vi "_Update Oscillators.vi"(4 "Pole In":bool[](array[boolean]), 5 "UpdateInput (F)":bool, 6 "ADC Array":i32[](array[numeric]), 7 "ADC Table":T1[](array[typedef]), 8 "Pole Swap (T)":bool=TRUE, 9 "Update (T)":bool=TRUE, 10 "Mode(pos)":bool=TRUE, 11 "Oscillator Settings":refnum<vi>) -> (1 "Q1RF Frequency":dbl, 3 "Pole":bool[](array[boolean]))   [LabVIEW 2012]
uses:
  Type/_RT Configuration 2.ctl
  Type/_RT Command.ctl
  Configuration/_Global Configuration.vi
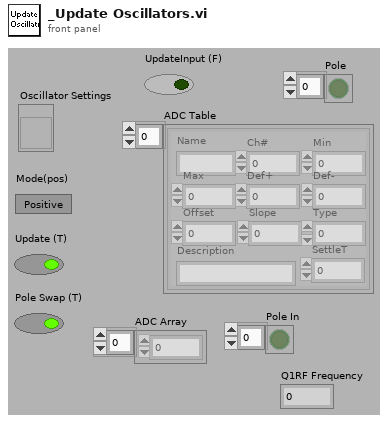
[diagram p1: front panel]
types:
  T1 = typedef "_RT Configuration 2.ctl" = cluster{"Name":string, "Ch#":u8, "Min":dbl, "Max":dbl, "Def+":dbl, "Def-":dbl, "Offset":dbl, "Slope":dbl, "Type":u8, "Description":string, "SettleT":dbl}
  T2 = typedef "_RT Instrument 2.ctl" = cluster{"Table":T1[], "Instrument":string[]}
  T3 = typedef "_RT Command.ctl" = enum16{"Start", "Stop", "Runtime Update", "Get Data", "Get Info", "Get Status", "Get Param", "Get Config", "Get Table", "Read ADC", "Set Oscillator", "Update Config", "Update Table", "Set All Pol", "Set Pol and DC", "Set Max Mass", "Toggle RP", "Toggle EL", "Set PIC", "Initialize Turbo", "Send Turbo Comm", "Close Turbo", "P1", "P2", "P3", "Send Serial", "Set LC Out", "Get LC In", "Read VAC", "Test Table", "Toggle Power", "Get Startup", "Set Startup", "Get ADC Table", "Set ADC Table", "Get Brief Status", "Get Detail Status", "Auxiliary Update", "Set CC Logics", "Set CC Input Logics", "Ignore Error"}
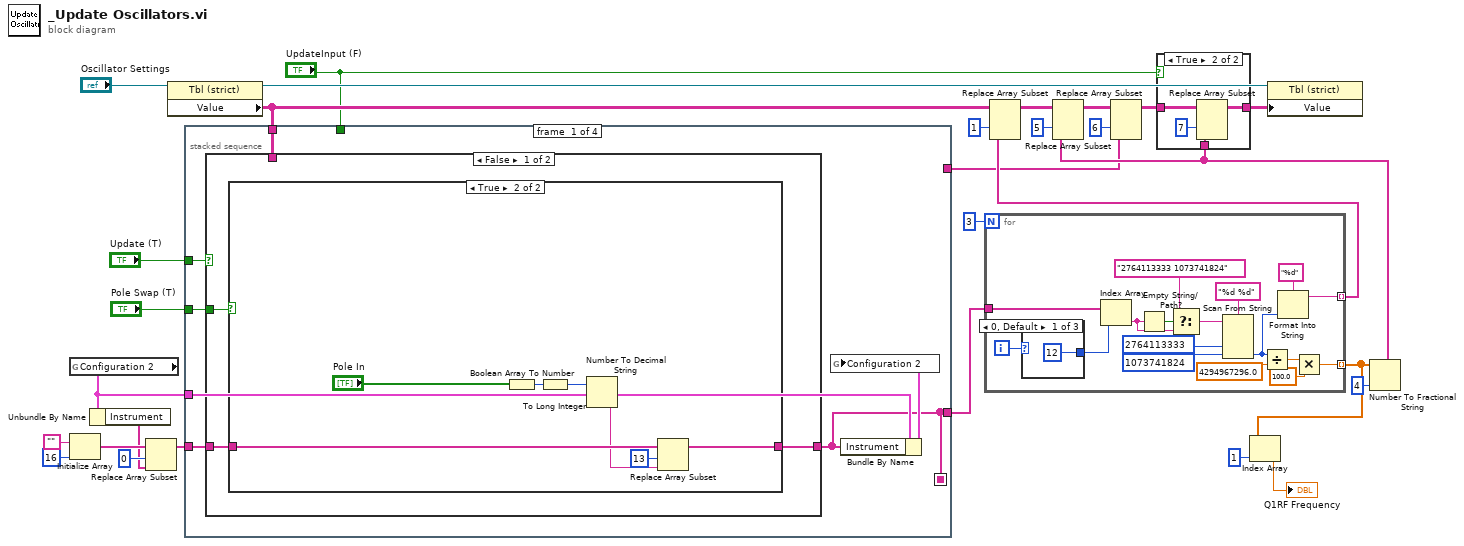
[diagram p0: block diagram]
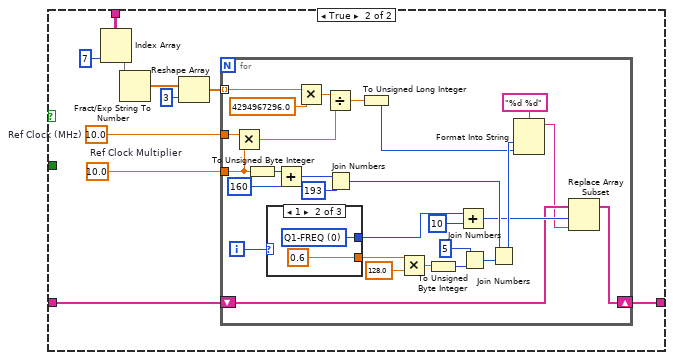
[diagram p4: hidden frame]
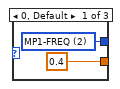
[diagram p5: hidden frame]
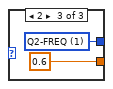
[diagram p6: hidden frame]
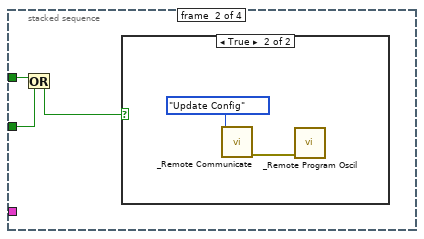
[diagram p7: hidden frame]
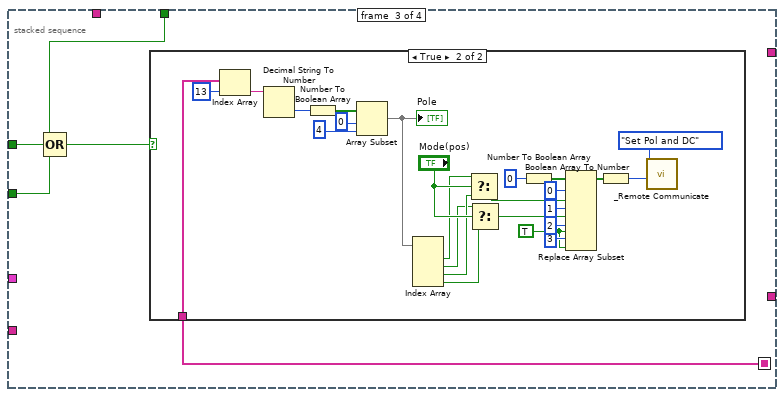
[diagram p9: hidden frame]
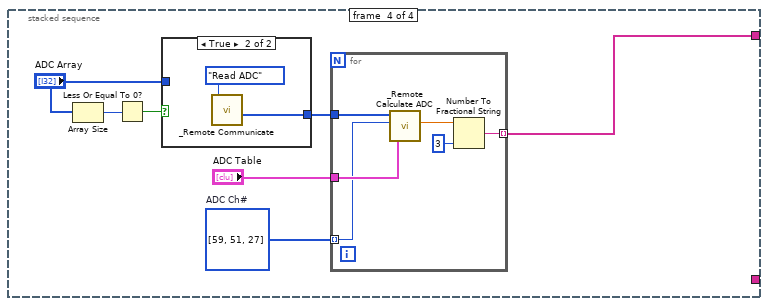
[diagram p11: hidden frame]
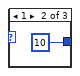
[diagram p13: hidden frame]
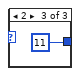
[diagram p14: hidden frame]
diagram:
  n1 = global read "_Global Configuration.vi" "Configuration 2"() -> (w22:T2)
  n2 = Initialize Array("", 16 ("dimension size")) -> (w26:string[])
  n3 = Unbundle By Name(w22) -> ("Instrument"=w24:string[])
  n4 = Replace Array Subset(array=w26, new element=w24, index=0) -> (w23:string[])
  n5 = property class="Tbl (strict)"(reference="Oscillator Settings") -> (reference out=w19:refnum<vi>, "Value"=w11:string[][])  [unwired: 1 in, 1 out]
  n6 = stacked-sequence {
    seq-local: [w30 _ _ _] -> [_ _ w101 _]
    tunnel: w11 -> [w36 _ _ _]
    tunnel: w23 -> [w35 _ _ _]
    tunnel: w22 -> [w33 _ _ _]
    tunnel: [w30 _ _ _] -> w13
    tunnel: "Update (T)" -> [w32 w94 w99 _]
    tunnel: "Pole Swap (T)" -> [w31 w93 w98 _]
    tunnel: [_ _ _ w130] -> w5
    tunnel: "UpdateInput (F)" -> [_ _ w100 _]
    frame #0 {
      n7 = case shown="False" w32 {
        tunnel: w36 -> [_ w57]
        tunnel: w35 -> [w39 w49]
        tunnel: [w37 w48] -> w30
        tunnel: w31 -> [w38 _]
        frame False {
          n8 = case shown="True" w38 {
            tunnel: w39 -> [w40 w45]
            tunnel: [w40 w44] -> w37
            frame False {
            }
            frame True {
              n9 = Boolean Array To Number(Boolean array="Pole In") -> (number=w46:u32)
              n10 = To Long Integer(number=w46) -> (32bit integer=w47:i32)
              n11 = Number To Decimal String(number=w47) -> (decimal integer string=w43:string)  [unwired: 1 out]
              n12 = Replace Array Subset(array=w45, new element=w43, index=13) -> (w44:string[])
            }
          }
        }
        frame True {
          w53 = 10.0  # Ref Clock Multiplier
          w54 = 10.0  # Ref Clock (MHz)
          n13 = Index Array(array=w57, index (col)=7 ("disabled index (col)")) -> (element=w55:string[])  [unwired: 1 in]
          n14 = Fract/Exp String To Number(string=w55) -> (number=w52:dbl[])  [unwired: 4 out]
          n15 = Reshape Array(w52, 3 ("dimension size")) -> (w51:dbl[])
          n16 = for {
            tunnel: w54 -> [w80]
            tunnel: w53 -> [w77]
            tunnel: w51 -> [w82] mode=indexing
            shift-right: [w58] -> w48
            shift-left: w49 -> [w60]
            i -> [w85]
            n17 = Multiply(x=w80, y=w77) -> (x*y=w79:dbl)
            n18 = To Unsigned Byte Integer(number=w77) -> (unsigned 8bit integer=w78:u8)
            n19 = case shown="1" w85 {
              tunnel: [w87 w89 w91] -> w62
              tunnel: [0.4 ("t") 0.6 ("t") 0.6 ("t")] -> w71
              frame 0, Default {
                w87 = u32 2 items=["Q1-FREQ", "Q2-FREQ", "MP1-FREQ"] ("Chip Select")
              }
              frame 1 {
                w89 = u32 0 items=["Q1-FREQ", "Q2-FREQ", "MP1-FREQ"] ("Chip Select")
              }
              frame 2 {
                w91 = u32 1 items=["Q1-FREQ", "Q2-FREQ", "MP1-FREQ"] ("Chip Select")
              }
            }
            n20 = Add(x=w78, y=u8 160) -> (x+y=w75:u8)
            n21 = Multiply(x=w82, y=4294967296.0) -> (x*y=w84:dbl)
            n22 = Divide(x=w84, y=w79) -> (x/y=w83:dbl)
            n23 = Join Numbers(hi=w75, lo=u8 193 ("Register 1")) -> ((hi.lo)=w67:u16)
            n24 = To Unsigned Long Integer(number=w83) -> (unsigned 32bit integer=w64:u32)
            n25 = Multiply(x=w71, y=128.0) -> (x*y=w72:dbl)
            n26 = To Unsigned Byte Integer(number=w72) -> (unsigned 8bit integer=w70:u8)
            n27 = Add(x=w62, y=u32 10) -> (x+y=w61:u32)
            n28 = Join Numbers(hi=u8 5 ("Register 6"), lo=w70) -> ((hi.lo)=w68:u16)
            n29 = Join Numbers(hi=w67, lo=w68) -> ((hi.lo)=w65:u32)
            n30 = Format Into String(format string="%d %d", w65, w64) -> (resulting string=w59:string)  [unwired: 2 in, 1 out]
            n31 = Replace Array Subset(array=w60, new element=w59, index=w61) -> (w58:string[])
          }
        }
      }
      n32 = Bundle By Name(cluster=w33, "Instrument"=w30) -> (w34:T2)
      n33 = global write "_Global Configuration.vi" "Configuration 2"(w34) -> ()
    }
    frame #1 {
      n34 = Or(x=w94, y=w93) -> (x .or. y?=w92:bool)
      n35 = case shown="True" w92 {
        frame False {
        }
        frame True {
          n36 = call "_Remote Communicate.vi"("Command"=_RT_Command."Update Config") -> ("error out"=w95:errorcluster)  [unwired: 5 in, 3 out]
          n37 = call "_Remote Program Oscil.vi"("error in (no error)"=w95) -> ()  [unwired: 1 out]
        }
      }
    }
    frame #2 {
      n38 = Compound Arithmetic op=OR(w100, w99, w98) -> (w97:bool)
      n39 = case shown="True" w97 {
        tunnel: w101 -> [_ w120]
        frame False {
        }
        frame True {
          w112 = TRUE ("new element/subarray")
          n40 = Index Array(array=w120, index=13) -> (element=w122:string)
          n41 = Decimal String To Number(string=w122) -> (number=w123:i32)  [unwired: 3 out]
          n42 = Number To Boolean Array(number=w123) -> (Boolean array=w124:bool[])
          n43 = Array Subset(array=w124, index=0, length=4) -> (w102:bool[])
          "Pole" <- w102
          n44 = Index Array(array=w102) -> (element #1=w108:bool, element #2=w104:bool, element #3=w107:bool, element #4=w106:bool)  [unwired: 4 in]
          n45 = Select(t=w108, s="Mode(pos)", f=w107) -> (s? t:f=w105:bool)
          n46 = Select(t=w104, s="Mode(pos)", f=w106) -> (s? t:f=w103:bool)
          n47 = Number To Boolean Array(number=u16 0) -> (Boolean array=w114:bool[])
          n48 = Replace Array Subset(array=w114, new element #1=w105, index #1=0 ("index"), new element #2=w103, index #2=1 ("index"), new element #3=w112, index #3=2 ("index"), new element #4=w112, index #4=3 ("index")) -> (w119:bool[])
          n49 = Boolean Array To Number(Boolean array=w119) -> (number=w110:u16)
          n50 = call "_Remote Communicate.vi"("DC Param"=w110, "Command"=_RT_Command."Set Pol and DC") -> ()  [unwired: 4 in, 4 out]
        }
      }
    }
    frame #3 {
      w133 = u8[] [59, 51, 27]  # ADC Ch#
      n51 = Array Size(array="ADC Array") -> (size(s)=w129:i32)
      n52 = Less Or Equal To 0?(x=w129) -> (x <= 0?=w128:bool)
      n53 = case shown="True" w128 {
        tunnel: [w134 w135] -> w132
        tunnel: "ADC Array" -> [w134 _]
        frame False {
        }
        frame True {
          n54 = call "_Remote Communicate.vi"("Command"=_RT_Command."Read ADC") -> ("Data Array"=w135:i32[])  [unwired: 5 in, 3 out]
        }
      }
      n55 = for {
        tunnel: w133 -> [w140] mode=indexing
        tunnel: w132 -> [w141]
        tunnel: "ADC Table" -> [w142]
        tunnel: [w137] -> w130 mode=indexing
        n56 = call "_Remote Calculate ADC.vi"("ADC Table"=w142, "ADC Channel (64)"=w140, "ADC Values"=w141) -> ("User Value"=w138:dbl)  [unwired: 1 in, 3 out]
        n57 = Number To Fractional String(number=w138, precision (6)=i16 3) -> (F-format string=w137:string)  [unwired: 2 out]
      }
    }
  }
  n58 = for {
    N: 3 -> [_]
    tunnel: w13 -> [w158]
    tunnel: [w146] -> w3 mode=indexing
    tunnel: [w143] -> w9 mode=indexing
    i -> [w159]
    n59 = case shown="0, Default" w159 {
      tunnel: [12 ("y") 10 ("y") 11 ("y")] -> w157
      frame 0, Default {
      }
      frame 1 {
      }
      frame 2 {
      }
    }
    n60 = Index Array(array=w158, index=w157) -> (element=w152:string)
    n61 = Empty String/Path?(string/path=w152) -> (empty?=w155:bool)
    n62 = Select(t="2764113333 1073741824", s=w155, f=w152) -> (s? t:f=w153:string)
    n63 = Scan From String(format string="%d %d", input string=w153, default 1=u32 2764113333 ("default value 1"), default 2=u32 1073741824 ("default value 1")) -> (output 2=w144:u32)  [unwired: 2 in, 4 out]
    n64 = Divide(x=w144, y=4294967296.0) -> (x/y=w148:dbl)
    n65 = Format Into String(format string="%d", w144) -> (resulting string=w143:string)  [unwired: 2 in, 1 out]
    n66 = Multiply(x=w148, y=100.0) -> (x*y=w146:dbl)
  }
  n67 = Replace Array Subset(array=w11, new element=w9, index (col)=1 ("disabled index (col)")) -> (w10:string[][])  [unwired: 1 in]
  n68 = Index Array(array=w3, index=1) -> (element=→"Q1RF Frequency":dbl)
  n69 = Number To Fractional String(number=w3, precision (6)=i16 4) -> (F-format string=w17:string[])  [unwired: 2 out]
  n70 = Replace Array Subset(array=w10, new element=w17, index (col)=5 ("disabled index (col)")) -> (w7:string[][])  [unwired: 1 in]
  n71 = Replace Array Subset(array=w7, new element=w5, index (col)=6 ("disabled index (col)")) -> (w6:string[][])  [unwired: 1 in]
  n72 = case shown="True" "UpdateInput (F)" {
    tunnel: w17 -> [_ w166]
    tunnel: [w163 w165] -> w16
    tunnel: w6 -> [w163 w164]
    frame False {
    }
    frame True {
      n73 = Replace Array Subset(array=w164, new element=w166, index (col)=7 ("disabled index (col)")) -> (w165:string[][])  [unwired: 1 in]
    }
  }
  n74 = property class="Tbl (strict)"(reference=w19, "Value"=w16) -> ()  [unwired: 1 in, 2 out]
